vi "ma_Spectrum Averaging (real) no State.vi"(6 "state info":T2 {"real spectrum" format="%0.2f"; "averages completed" format="%0.2f"; "df" format="%0.2f"; "complex spectrum" format="%0.2f"; "spectrum parameters"."window" items=["Rectangle"=0, "Hanning"=1, "Hamming"=2, "Blackman-Harris"=3, "Exact Blackman"=4, "Blackman"=5, "Flat Top"=6, "4 Term B-Harris "=7, "7 Term B-Harris"=8, "Low Sidelobe"=9, "Blackman Nuttall"=11, "Triangle"=30, "Bartlett-Hanning"=31, "Bohman"=32, "Parzen"=33, "Welch"=34, "Kaiser"=60, "Dolph-Chebyshev"=61, "Gaussian"=62]; "dt" format="%0.2f"; "timestamp" format="%0.2f"; "dt history" format="%0.2f"; "t0 history" format="%0.2f"}, 7 "retrieve last spectrum (F)":bool, 8 "restart averaging (F)":bool, 9 "averaging parameters":T3={"averaging mode"=enum."No averaging", "weighting mode"=enum."Exponential", "number of averages"=10} {"number of averages" min=1}, 10 "df":dbl format="%0.2f", 11 "real spectrum":dbl[](array[numeric]) format="%0.2f") -> (0 "averages completed":dbl format="%0.2f", 1 "averaging done":bool, 2 "df":dbl format="%0.2f", 3 "averaged real spectrum":dbl[](array[numeric]) format="%0.2f", 4 "state info":T2 {"real spectrum" format="%0.2f"; "averages completed" format="%0.2f"; "df" format="%0.2f"; "complex spectrum" format="%0.2f"; "spectrum parameters"."window" items=["Rectangle"=0, "Hanning"=1, "Hamming"=2, "Blackman-Harris"=3, "Exact Blackman"=4, "Blackman"=5, "Flat Top"=6, "4 Term B-Harris "=7, "7 Term B-Harris"=8, "Low Sidelobe"=9, "Blackman Nuttall"=11, "Triangle"=30, "Bartlett-Hanning"=31, "Bohman"=32, "Parzen"=33, "Welch"=34, "Kaiser"=60, "Dolph-Chebyshev"=61, "Gaussian"=62]; "dt" format="%0.2f"; "timestamp" format="%0.2f"; "dt history" format="%0.2f"; "t0 history" format="%0.2f"})   [LabVIEW 2020, in "NI_MAPro.lvlib"]
uses:
  NI_MAPro.lvlib
  windowTd.ctl
  NI_AALPro.lvlib
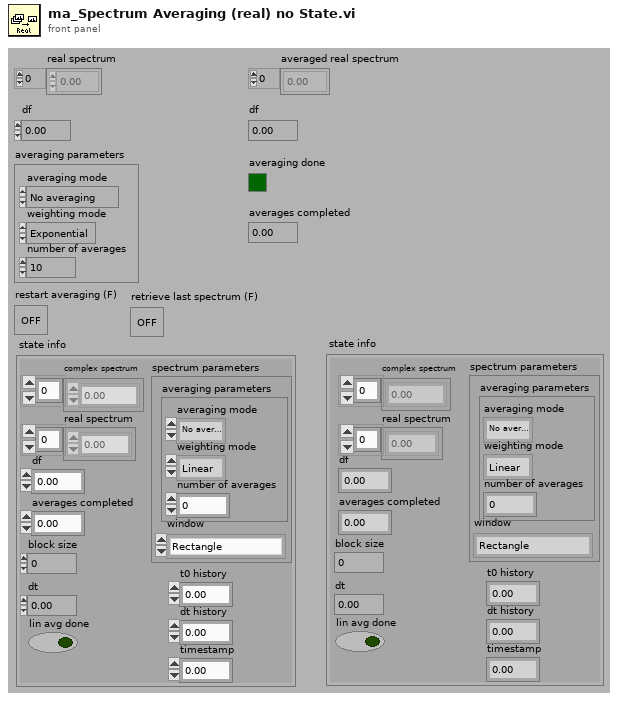
[diagram p1: front panel]
types:
  T1 = typedef "NI_AALPro.lvlib/windowTd.ctl" = u32
  T2 = cluster{"block size":i32, "dt":dbl, "spectrum parameters":cluster{"averaging parameters":cluster{"averaging mode":enum16{"No averaging", "Vector averaging", "RMS averaging", "Peak hold"}, "weighting mode":enum16{"Linear", "Exponential"}, "number of averages":u32}, "window":T1}, "df":dbl, "averages completed":dbl, "complex spectrum":cdb[], "real spectrum":dbl[], "t0 history":dbl, "dt history":dbl, "timestamp":dbl, "lin avg done":bool}
  T3 = cluster{"averaging mode":enum16{"No averaging", "Vector averaging", "RMS averaging", "Peak hold"}, "weighting mode":enum16{"Linear", "Exponential"}, "number of averages":u32}
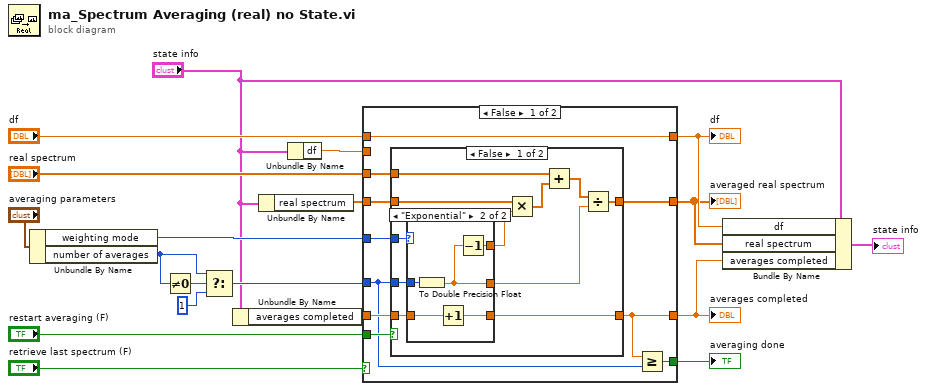
[diagram p0: block diagram]
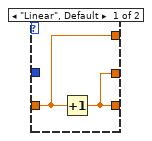
[diagram p2: hidden frame]
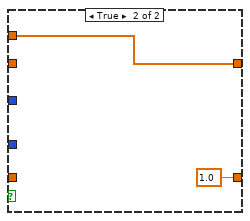
[diagram p3: hidden frame]
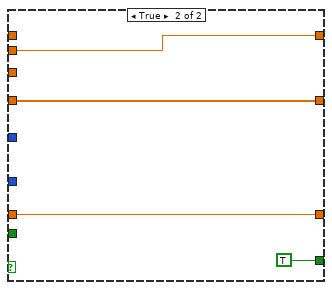
[diagram p4: hidden frame]
diagram:
  n1 = Unbundle By Name("averaging parameters") -> ("weighting mode"=w16:enum16{"Linear", "Exponential"}, "number of averages"=w9:u32)
  n2 = Not Equal To 0?(x=w9) -> (x != 0?=w12:bool)
  n3 = Select(t=w9, s=w12, f=u32 1) -> (s? t:f=w10:u32)
  n4 = Unbundle By Name("state info") -> ("averages completed"=w6:dbl)
  n5 = Unbundle By Name("state info") -> ("real spectrum"=w8:dbl[])
  n6 = Unbundle By Name("state info") -> ("df"=w7:dbl)
  n7 = case shown="False" "retrieve last spectrum (F)" {
    tunnel: [w29 w53] -> w4
    tunnel: w6 -> [w28 w52]
    tunnel: w8 -> [w27 w53]
    tunnel: w16 -> [w26 _]
    tunnel: "real spectrum" -> [w25 _]
    tunnel: "restart averaging (F)" -> [w24 _]
    tunnel: [w23 w52] -> w3
    tunnel: w10 -> [w22 _]
    tunnel: [w21 TRUE] -> w15
    tunnel: "df" -> [w20 _]
    tunnel: [w20 w50] -> w5
    tunnel: w7 -> [_ w50]
    frame False {
      n8 = case shown="False" w24 {
        tunnel: [w37 w48] -> w29
        tunnel: [w32 1.0] -> w23
        tunnel: w28 -> [w35 _]
        tunnel: w27 -> [w40 _]
        tunnel: w25 -> [w36 w48]
        tunnel: w26 -> [w33 _]
        tunnel: w22 -> [w30 _]
        frame False {
          n9 = case shown="\"Exponential\"" w33 {
            tunnel: w35 -> [w42 w46]
            tunnel: [w41 w47] -> w32
            tunnel: [w42 w43] -> w34
            tunnel: [w41 w44] -> w31
            tunnel: w30 -> [_ w45]
            frame "Linear", Default {
              n10 = Increment(x=w42) -> (x+1=w41:dbl)
            }
            frame "Exponential" {
              n11 = To Double Precision Float(number=w45) -> (double precision float=w44:dbl)
              n12 = Increment(x=w46) -> (x+1=w47:dbl)
              n13 = Decrement(x=w44) -> (x-1=w43:dbl)
            }
          }
          n14 = Multiply(x=w40, y=w34) -> (x*y=w39:dbl[])
          n15 = Add(x=w36, y=w39) -> (x+y=w38:dbl[])
          n16 = Divide(x=w38, y=w31) -> (x/y=w37:dbl[])
        }
        frame True {
        }
      }
      n17 = Greater Or Equal?(x=w23, y=w22) -> (x >= y?=w21:bool)
    }
    frame True {
    }
  }
  "averaged real spectrum" <- w4
  "averages completed" <- w3
  "averaging done" <- w15
  "df" <- w5
  n18 = Bundle By Name(cluster="state info", "df"=w5, "real spectrum"=w4, "averages completed"=w3) -> (→"state info":T2)
